vi "Watchdog_Functional_Global.vi"(7 "Watchdog":T1, 11 "error in":errorcluster) -> (2 "Elapsed":string, 3 "error out":errorcluster, 5 "Elapsed":i32[](array[numeric]))   [LabVIEW 2018]
uses:
  Controls/Enums/WatchdogTimer_Enum.ctl
  Controls/Clusts/WatchdogTimer_Clust.ctl
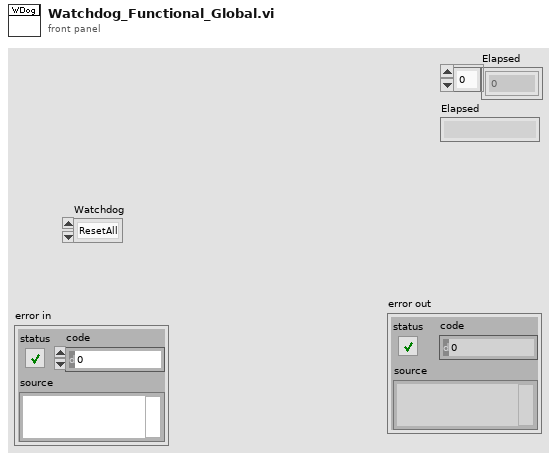
[diagram p1: front panel]
types:
  T1 = typedef "WatchdogTimer_Enum.ctl" = enum16{"ResetAll", "CheckAll", "HW1", "HW2", "Tones", "FP", "Noise", "Log", "TCP", "AI", "TC", "ADAM", "Disdrom", "TE", "Weather"}
  T2 = typedef "WatchdogTimer_Clust.ctl" = cluster{"HW1":i32, "HW2":i32, "Tones":i32, "FP":i32, "Noise":i32, "Log":i32, "TCP":i32, "AI":i32, "TC":i32, "ADAM":i32, "Disdrom":i32, "TE":i32, "Weather":i32}
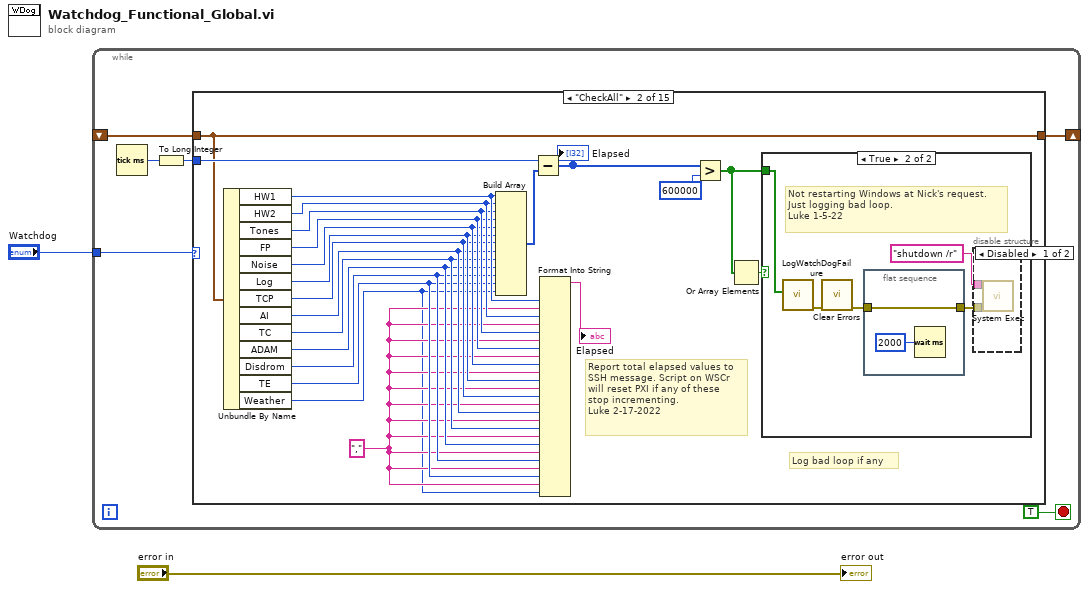
[diagram p0: block diagram]
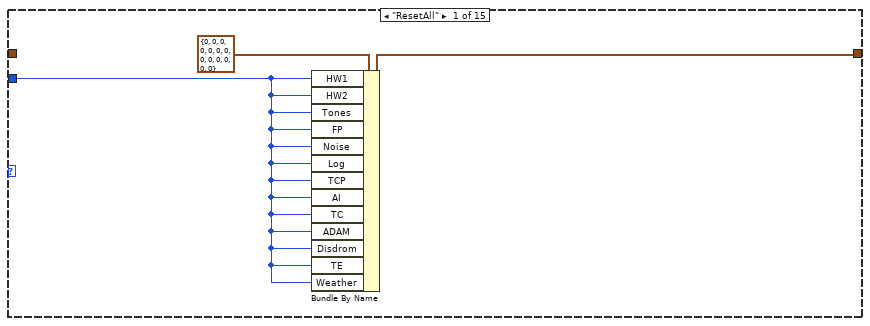
[diagram p2: hidden frame]
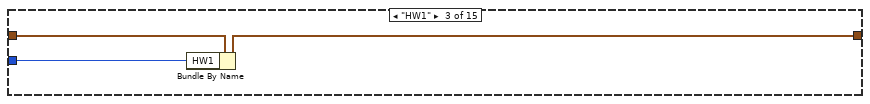
[diagram p5: hidden frame]
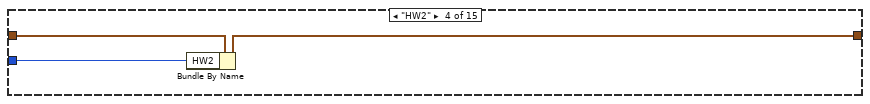
[diagram p6: hidden frame]
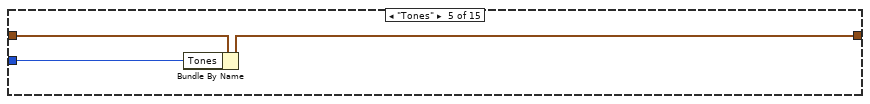
[diagram p7: hidden frame]
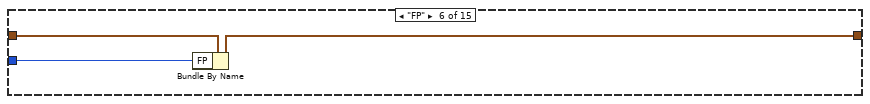
[diagram p8: hidden frame]
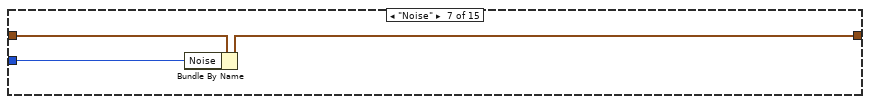
[diagram p9: hidden frame]
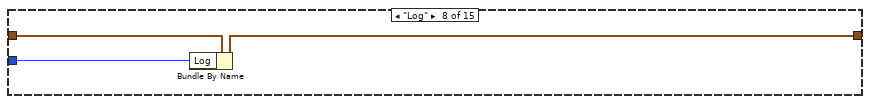
[diagram p10: hidden frame]
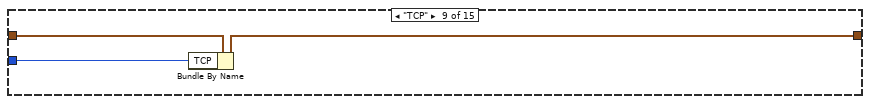
[diagram p11: hidden frame]
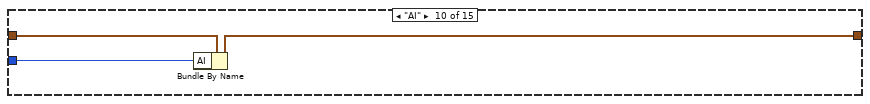
[diagram p12: hidden frame]
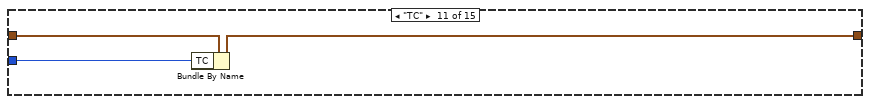
[diagram p13: hidden frame]
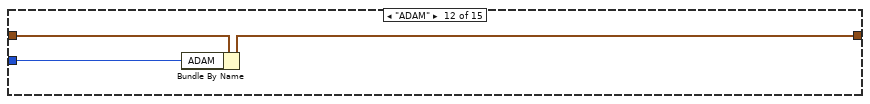
[diagram p14: hidden frame]
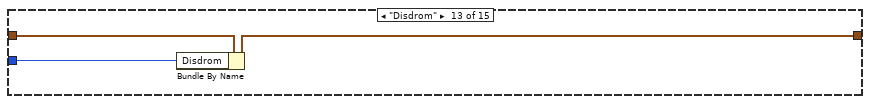
[diagram p15: hidden frame]
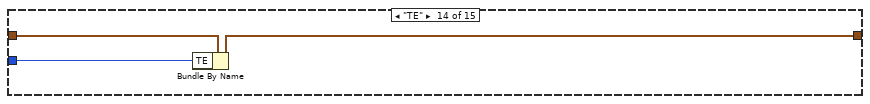
[diagram p16: hidden frame]
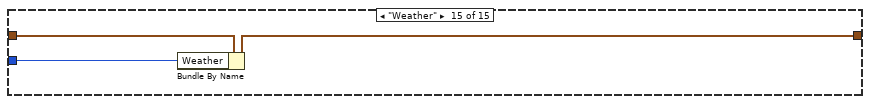
[diagram p17: hidden frame]
diagram:
  n1 = while {
    tunnel: "Watchdog" -> [w8]
    shift-right: [w6] -> _
    shift-left: _ -> [w7]
    stop <- TRUE stop-if-true
    n2 = Tick Count (ms)() -> (millisecond timer value=w5:u32)
    n3 = To Long Integer(number=w5) -> (32bit integer=w4:i32)
    n4 = case shown="\"CheckAll\"" w8 {
      tunnel: w7 -> [_ w32 w45 w48 w51 w54 w57 w60 w63 w66 w69 w72 w75 w78 w81]
      tunnel: [w10 w32 w44 w47 w50 w53 w56 w59 w62 w65 w68 w71 w74 w77 w80] -> w6
      tunnel: w4 -> [w9 w33 w43 w46 w49 w52 w55 w58 w61 w64 w67 w70 w73 w76 w79]
      frame "ResetAll" {
        n5 = Bundle By Name(cluster=T2 {"HW1"=0, "HW2"=0, "Tones"=0, "FP"=0, "Noise"=0, "Log"=0, "TCP"=0, "AI"=0, "TC"=0, "ADAM"=0, "Disdrom"=0, "TE"=0, "Weather"=0}, "HW1"=w9, "HW2"=w9, "Tones"=w9, "FP"=w9, "Noise"=w9, "Log"=w9, "TCP"=w9, "AI"=w9, "TC"=w9, "ADAM"=w9, "Disdrom"=w9, "TE"=w9, "Weather"=w9) -> (w10:T2)
      }
      frame "CheckAll" {
        w16 = ","
        # "Log bad loop if any"
        # "Report total elapsed values to \nSSH message. Script on WSCr\nwill reset PXI if any of these \nstop incrementing.\nLuke 2-17-2022"
        n6 = Unbundle By Name(w32) -> ("HW1"=w28:i32, "HW2"=w27:i32, "Tones"=w26:i32, "FP"=w25:i32, "Noise"=w24:i32, "Log"=w23:i32, "TCP"=w22:i32, "AI"=w21:i32, "TC"=w20:i32, "ADAM"=w19:i32, "Disdrom"=w18:i32, "TE"=w17:i32, "Weather"=w15:i32)
        n7 = Build Array(w28, w27, w26, w25, w24, w23, w22, w21, w20, w19, w18, w17, w15) -> (w13:i32[])
        n8 = Subtract(x=w33, y=w13) -> (x-y=w12:i32[])
        "Elapsed" <- w12
        n9 = Format Into String(w28, w16, w27, w16, w26, w16, w25, w16, w24, w16, w23, w16, w22, w16, w21, w16, w20, w16, w19, w16, w18, w16, w17, w16, w15) -> (resulting string=→"Elapsed":string)  [unwired: 3 in, 1 out]
        n10 = Greater?(x=w12, y=600000) -> (0:w29:bool[])
        n11 = Or Array Elements(Boolean array=w29) -> (logical OR=w30:bool)
        n12 = case shown="True" w30 {
          tunnel: w29 -> [_ w34]
          frame False {
          }
          frame True {
            # "Not restarting Windows at Nick's request.\nJust logging bad loop.\nLuke 1-5-22"
            n13 = call "LogWatchDogFailure.vi"("Elapsed"=w34) -> ("error out"=w38:errorcluster)  [unwired: 10 in]
            n14 = call <vilib>:"Clear Errors.vi"("error in (no error)"=w38) -> ("error out"=w35:errorcluster)  [unwired: 5 in, 1 out]
            n15 = flat-sequence {
              tunnel: [w41] -> w36
              tunnel: w35 -> [w41]
              frame #0 {
                n16 = Wait (ms)(milliseconds to wait=u32 2000) -> ()  [unwired: 1 out]
              }
            }
            n17 = disable-structure shown="Disabled" {
              disable-tunnel: "shutdown /r" ("command line") -> [w40 _]
              disable-tunnel: w36 -> [w39 _]
              frame Disabled {
                n18 = call <vilib>:"System Exec.vi"("error in (no error)"=w39, "command line"=w40) -> ()  [unwired: 6 in, 4 out]
              }
              frame Enabled {
              }
            }
          }
        }
      }
      frame "HW1" {
        n19 = Bundle By Name(cluster=w45, "HW1"=w43) -> (w44:T2)
      }
      frame "HW2" {
        n20 = Bundle By Name(cluster=w48, "HW2"=w46) -> (w47:T2)
      }
      frame "Tones" {
        n21 = Bundle By Name(cluster=w51, "Tones"=w49) -> (w50:T2)
      }
      frame "FP" {
        n22 = Bundle By Name(cluster=w54, "FP"=w52) -> (w53:T2)
      }
      frame "Noise" {
        n23 = Bundle By Name(cluster=w57, "Noise"=w55) -> (w56:T2)
      }
      frame "Log" {
        n24 = Bundle By Name(cluster=w60, "Log"=w58) -> (w59:T2)
      }
      frame "TCP" {
        n25 = Bundle By Name(cluster=w63, "TCP"=w61) -> (w62:T2)
      }
      frame "AI" {
        n26 = Bundle By Name(cluster=w66, "AI"=w64) -> (w65:T2)
      }
      frame "TC" {
        n27 = Bundle By Name(cluster=w69, "TC"=w67) -> (w68:T2)
      }
      frame "ADAM" {
        n28 = Bundle By Name(cluster=w72, "ADAM"=w70) -> (w71:T2)
      }
      frame "Disdrom" {
        n29 = Bundle By Name(cluster=w75, "Disdrom"=w73) -> (w74:T2)
      }
      frame "TE" {
        n30 = Bundle By Name(cluster=w78, "TE"=w76) -> (w77:T2)
      }
      frame "Weather" {
        n31 = Bundle By Name(cluster=w81, "Weather"=w79) -> (w80:T2)
      }
    }
  }
  "error out" <- "error in"
